vi "PV ActiveLine - Time.vi"(7 "W/R":bool, 8 "Fehler (Eingang)":errorcluster, 9 "Minutes":i8=1 min=0 max=59 format="%02.0f", 10 "Hours":i8=1 min=0 max=23 format="%02.0f", 11 "Referenz in":refnum<visa-resource-name>) -> (0 "Cluster (Ausgang)":errorcluster, 1 "Minutes out":i8=1 min=1 max=12 format="%02.0f", 2 "Hours out":i8=1 min=1 max=31 format="%02.0f", 3 "Referenz out":refnum<visa-resource-name>)   [LabVIEW 2013, in "PV ActiveLine.lvlib"]
doc: "TIM - Time\n\nTransmit: TIM [,hh:mm]\nReceive: hh:mm\n\nhh:mm = Current time in the format hh:mm [24 h]"
uses:
  <instrlib>/PV ActiveLine/PV ActiveLine.lvlib
panel:
  # "Time to set"
  # "Time on device"
  # ":"
  # ":"
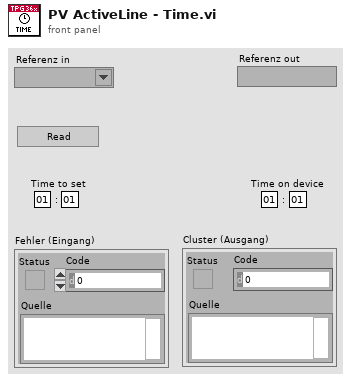
[diagram p1: front panel]
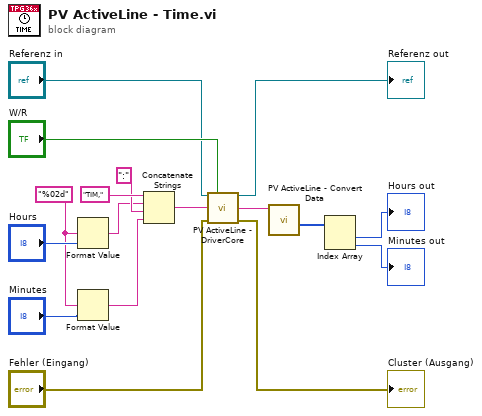
[diagram p0: block diagram]
diagram:
  w9 = "%02d" ("format string")
  n1 = Format Value(format string=w9, value (0)="Hours") -> (output string=w7:string)  [unwired: 1 in]
  n2 = Format Value(format string=w9, value (0)="Minutes") -> (output string=w8:string)  [unwired: 1 in]
  n3 = Concatenate Strings("TIM,", w7, ":" ("string"), w8) -> (w15:string)
  n4 = call <instrlib>:"PV ActiveLine - DriverCore.vi"("Referenz in"="Referenz in", "Write/Read"="W/R", "Command"=w15, "Fehler (Eingang)"="Fehler (Eingang)") -> ("Referenz out"=→"Referenz out":refnum<visa-resource-name>, "String Out"=w4:string, "Cluster (Ausgang)"=→"Cluster (Ausgang)":errorcluster)  [unwired: 9 in]
  n5 = call <instrlib>:"PV ActiveLine - Convert Data.vi"("String in"=w4) -> ("Integer Out"=w3:i32[])  [unwired: 7 in, 3 out]
  n6 = Index Array(array=w3) -> (element #1=→"Hours out":i32, element #2=→"Minutes out":i32)  [unwired: 2 in]
